vi "connect.vi"() -> ()   [LabVIEW 2013]
uses:
  <vilib>/httpClient/ClientHandle.ctl
  Controls/ConnectResponse.ctl
  <vilib>/httpClient/LabVIEWHTTPClient.lvlib
  <vilib>/wsapi/NI_WebServices.lvlib
panel:
  in  "unescaped string in":string
  out "WSurl":string
  out "value":T1
  out "client handle out":T2
  out "headers":string
  out "body":string
  out "error out":errorcluster
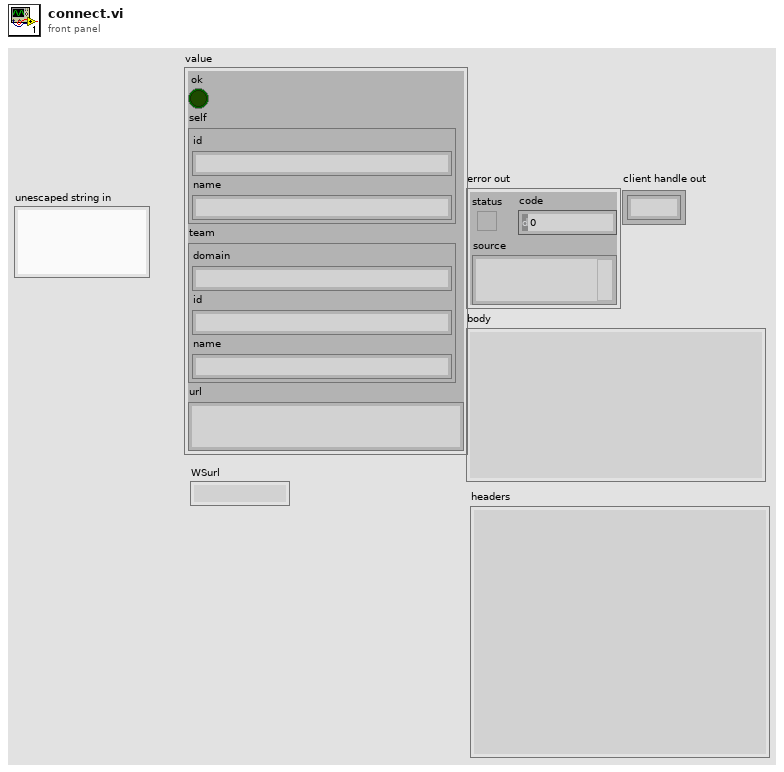
[diagram p1: front panel]
types:
  T1 = typedef "ConnectResponse.ctl" = cluster{"ok":bool, "self":cluster{"id":string, "name":string}, "team":cluster{"domain":string, "id":string, "name":string}, "url":string}
  T2 = typedef "LabVIEWHTTPClient.lvlib/ClientHandle.ctl" = refnum<k1>
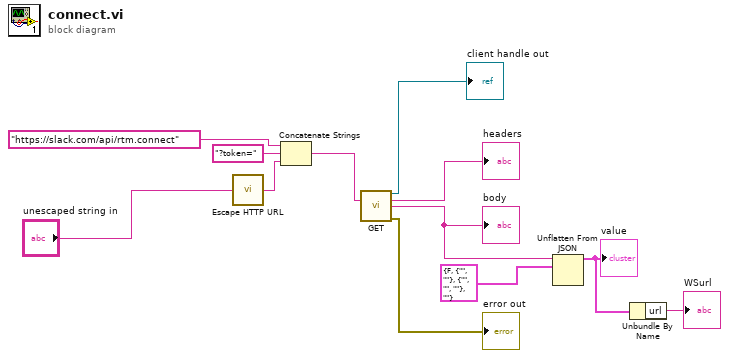
[diagram p0: block diagram]
diagram:
  n1 = call <vilib>:"Escape HTTP URL.vi"("unescaped string in"="unescaped string in") -> ("escaped string out"=w9:string)
  n2 = Concatenate Strings("https://slack.com/api/rtm.connect" ("url"), "?token=" ("string"), w9) -> (w6:string)
  n3 = call <vilib>:"GET.vi"("url"=w6) -> ("client handle out"=→"client handle out":T2, "headers"=→"headers":string, "body"=w5:string, "error out"=→"error out":errorcluster)  [unwired: 11 in]
  "body" <- w5
  n4 = Unflatten From JSON(JSON string=w5, type and defaults=T1 {"ok"=FALSE, "self"={"id"="", "name"=""}, "team"={"domain"="", "id"="", "name"=""}, "url"=""} ("Cluster")) -> (value=w3:T1)  [unwired: 5 in, 1 out]
  "value" <- w3
  n5 = Unbundle By Name(w3) -> ("url"=→"WSurl":string)
